vi "VI_CmdPrompt.vi"(7 "Mode":T2, 8 "error in (no error)":errorcluster, 9 "Activate?":bool=TRUE, 10 "communication_data":T1, 11 "STR_CmdPrompt_Ref":refnum<vi>) -> (0 "error out":errorcluster)   [LabVIEW 2020]
uses:
  TypeDefs/Enum_CmdPromptActions.ctl
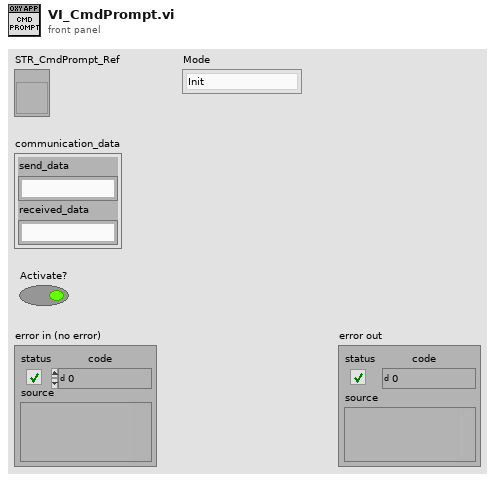
[diagram p1: front panel]
types:
  T1 = cluster{"send_data":string, "received_data":string}
  T2 = typedef "Enum_CmdPromptActions.ctl" = enum16{"Init", "Add", "EditSettings", "Close"}
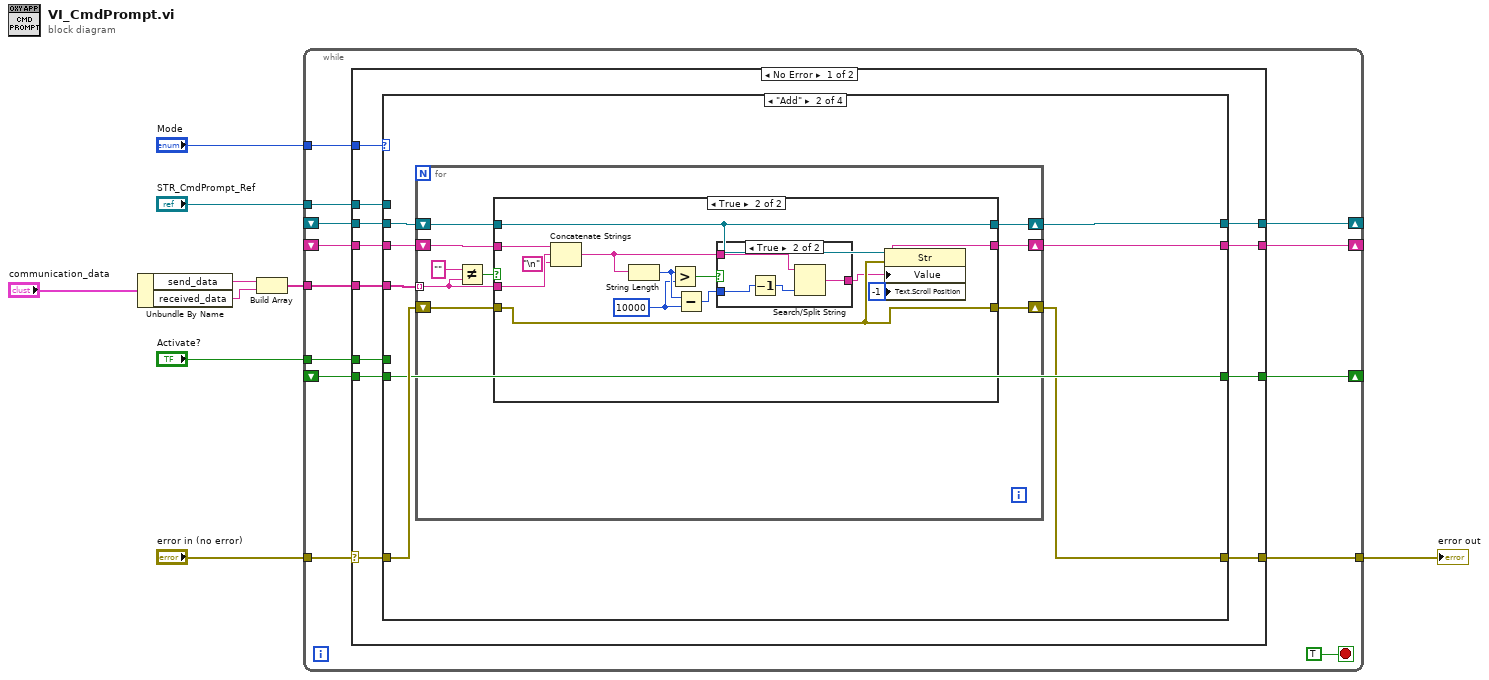
[diagram p0: block diagram]
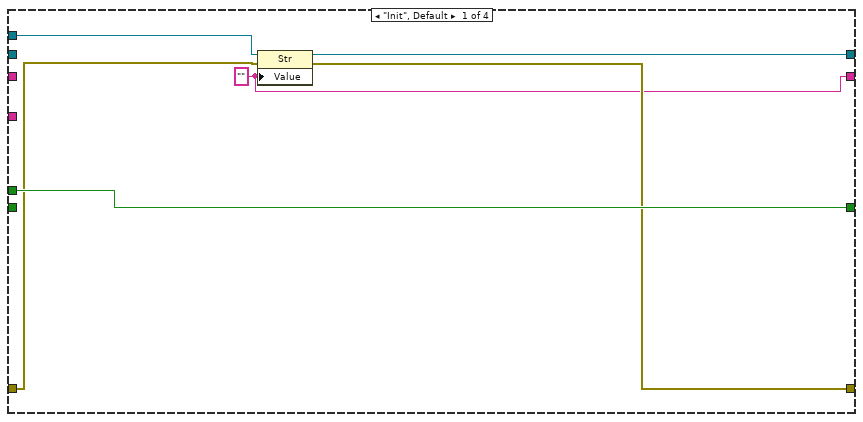
[diagram p2: hidden frame]
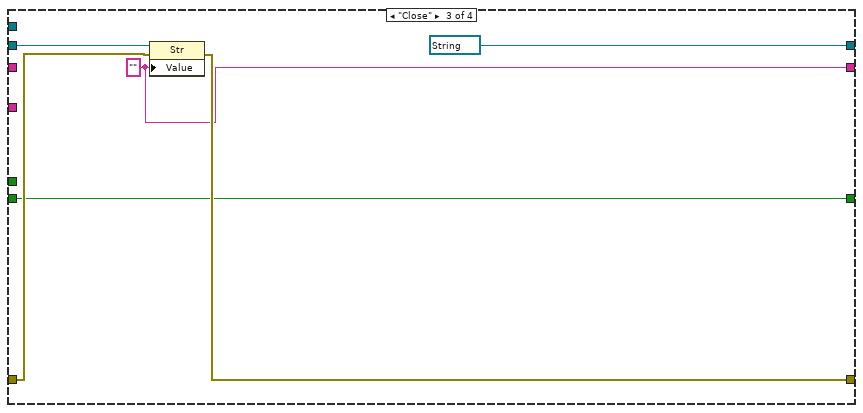
[diagram p5: hidden frame]
diagram:
  n1 = Unbundle By Name("communication_data") -> ("send_data"=w4:string, "received_data"=w3:string)
  n2 = Build Array(w4, w3) -> (w2:string[])
  n3 = while {
    tunnel: "Mode" -> [w22]
    tunnel: [w21] -> w7
    tunnel: "error in (no error)" -> [w16]
    shift-right: [w18] -> _
    shift-left: _ -> [w19]
    tunnel: w2 -> [w17]
    shift-right: [w14] -> _
    shift-left: _ -> [w15]
    tunnel: "STR_CmdPrompt_Ref" -> [w13]
    tunnel: "Activate?" -> [w12]
    shift-right: [w11] -> _
    shift-left: _ -> [w10]
    stop <- TRUE stop-if-true
    n4 = case shown="No Error" w16 {
      selector: w16 -> [w29 w89]
      tunnel: w22 -> [w34 _]
      tunnel: [w33 w89] -> w21
      tunnel: w19 -> [w32 w91]
      tunnel: [w31 w91] -> w18
      tunnel: w17 -> [w30 _]
      tunnel: w15 -> [w28 w90]
      tunnel: [w27 w90] -> w14
      tunnel: w13 -> [w26 _]
      tunnel: w12 -> [w25 _]
      tunnel: [w24 w88] -> w11
      tunnel: w10 -> [w23 w88]
      frame No Error {
        n5 = case shown="\"Add\"" w34 {
          tunnel: [w36 w41 w80 w85] -> w33
          tunnel: w29 -> [w37 w47 w81 w85]
          tunnel: w32 -> [_ w48 w82 w86]
          tunnel: [w39 w42 refnum<vi> refnum ("STR_CmdPrompt_Ref") w86] -> w31
          tunnel: w30 -> [_ w45 _ _]
          tunnel: w28 -> [_ w46 w79 w87]
          tunnel: [w40 w46 w79 w87] -> w27
          tunnel: w26 -> [w38 _ _ _]
          tunnel: w25 -> [w40 _ _ _]
          tunnel: [w35 w43 w78 w84] -> w24
          tunnel: w23 -> [_ w44 _ w84]
          frame "Init", Default {
            w35 = "" ("Value")
            n6 = property class="Str"(reference=w38, error in=w37, "Value"=w35) -> (reference out=w39:refnum<vi>, error out=w36:errorcluster)
          }
          frame "Add" {
            n7 = for {
              tunnel: w45 -> [w53] mode=indexing
              shift-right: [w55] -> w41
              shift-left: w47 -> [w54]
              shift-right: [w56] -> w42
              shift-left: w48 -> [w57]
              shift-right: [w50] -> w43
              shift-left: w44 -> [w49]
              n8 = Not Equal?(x="", y=w53) -> (x != y?=w52:bool)
              n9 = case shown="True" w52 {
                tunnel: w57 -> [w59 w64]
                tunnel: [w59 w64] -> w56
                tunnel: [w60 w63] -> w55
                tunnel: w54 -> [w60 w63]
                tunnel: w53 -> [_ w72]
                tunnel: [w58 w62] -> w50
                tunnel: w49 -> [w58 w65]
                frame False {
                }
                frame True {
                  w67 = 10000 ("y")
                  n10 = Concatenate Strings(w65, w72, "\n") -> (w70:string)
                  n11 = String Length(string=w70) -> (length=w68:i32)
                  n12 = Greater?(x=w68, y=w67) -> (0:w69:bool)
                  n13 = Subtract(x=w68, y=w67) -> (x-y=w66:i32)
                  n14 = case shown="True" w69 {
                    tunnel: [w73 w74] -> w62
                    tunnel: w70 -> [w73 w76]
                    tunnel: w66 -> [_ w77]
                    frame False {
                    }
                    frame True {
                      n15 = Decrement(x=w77) -> (x-1=w75:i32)
                      n16 = Search/Split String(string=w76, offset (0)=w75) -> (match + rest of string=w74:string)  [unwired: 1 in, 2 out]
                    }
                  }
                  n17 = property class="Str"(reference=w64, error in=w63, "Value"=w62, "Text.Scroll Position"=-1) -> ()  [unwired: 2 out]
                }
              }
            }
          }
          frame "Close" {
            w78 = "" ("Value")
            n18 = property class="Str"(reference=w82, error in=w81, "Value"=w78) -> (error out=w80:errorcluster)  [unwired: 1 out]
          }
          frame "EditSettings" {
          }
        }
      }
      frame Error {
      }
    }
  }
  "error out" <- w7
